vi "Barcode read.vi"(8 "error in":errorcluster, 11 "queue in":refnum<queue>) -> (0 "error out":errorcluster, 1 "exit":bool, 2 "read buffer":string, 3 "queue Out 2":refnum<queue>, 4 "Barcode Scan Bit":bool)   [LabVIEW 2015]
uses:
  Test  enqueue/AutoTest seq.ctl
  <vilib>/Utility/error.llb/whitespace.ctl
  <vilib>/Instr/_visa.llb/VISA Configure Serial Port (Instr).vi
  Galobal variable_TI.vi
  Project Setup/Globle Variable/GR_Servo.vi
panel:
  out "x = y?":bool
  out "substring":string
  out "error out 2":errorcluster
  out "error out":errorcluster
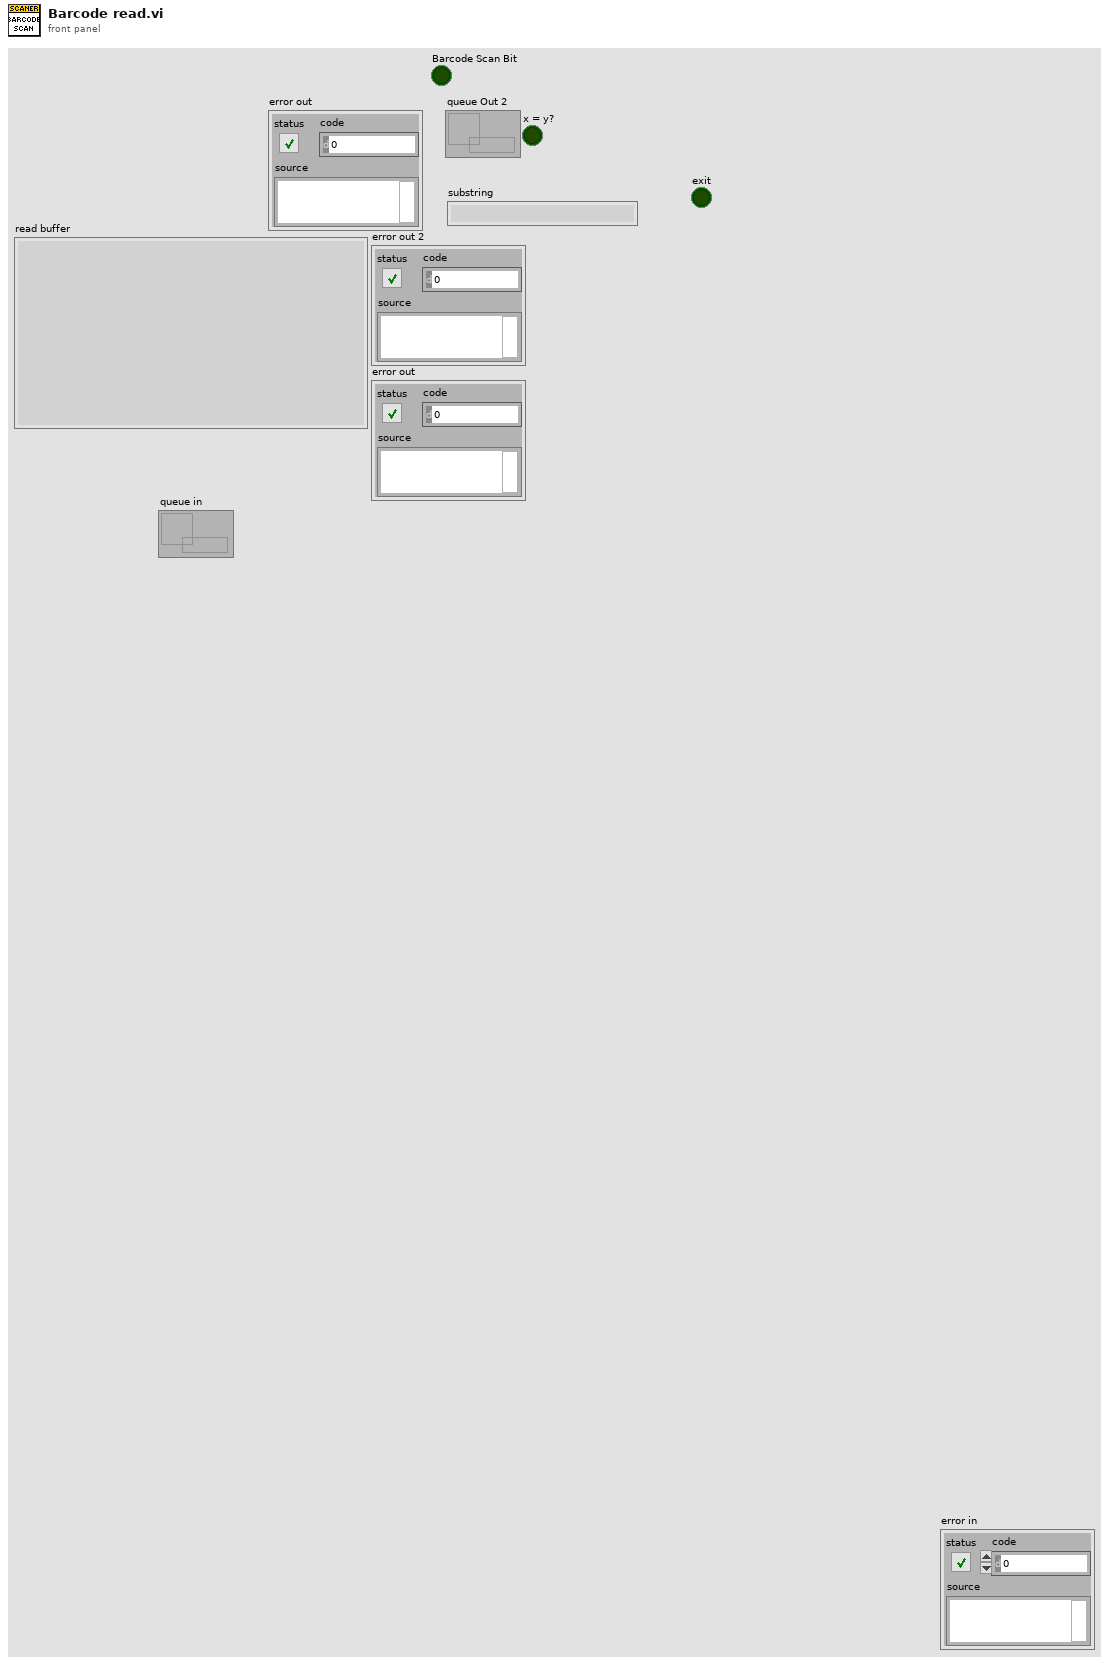
[diagram p1: front panel]
types:
  T1 = typedef "whitespace.ctl" = u16
  T2 = cluster{"MaxLoad(N) ":dbl, "Min Load(N)":dbl, "Load Offset":dbl, "Model":string, "MIC Code":string, "Dial Speedo":string, "Dial RMP":string, "Blinker":string, "Telltale":string}
  T3 = cluster{"Start":bool, "Emergency ":bool, "Reset":bool, "Home":bool, "Safety":bool}
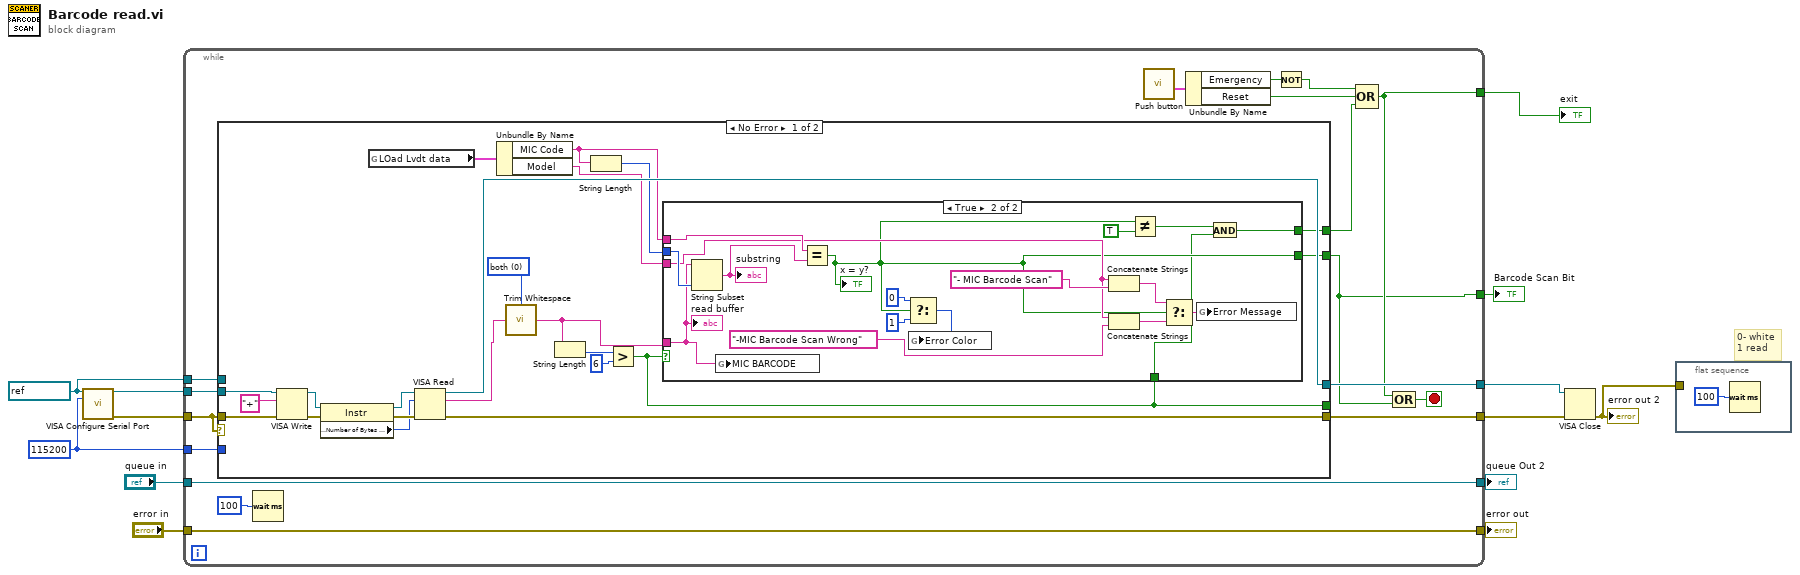
[diagram p0: block diagram]
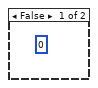
[diagram p2: hidden frame]
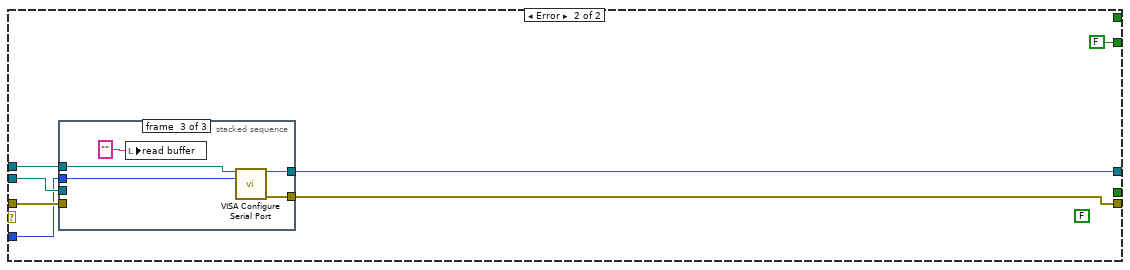
[diagram p3: hidden frame]
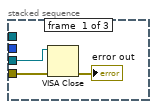
[diagram p4: hidden frame]
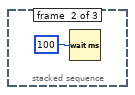
[diagram p5: hidden frame]
diagram:
  w8 = u32 115200 ("baud rate (9600)")
  w9 = refnum<visa-resource-name> "COM1" ("VISA resource name")
  # "0- white\n1 read"
  n1 = call-poly "VISA Configure Serial Port"("VISA resource name"=w9, "baud rate (9600)"=w8) -> ("VISA resource name out"=w13:refnum<visa-resource-name>, "error out"=w12:errorcluster)  [unwired: 12 in]
  n2 = while {
    tunnel: w13 -> [w30]
    tunnel: w12 -> [w28]
    tunnel: [w17] -> w11
    tunnel: [w29] -> w10
    tunnel: w9 -> [w27]
    tunnel: w8 -> [w26]
    tunnel: [w15] -> w7
    tunnel: [w23] -> w5
    tunnel: "queue in" -> [w23]
    tunnel: "error in" -> [w22]
    tunnel: [w22] -> w3
    tunnel: [w14] -> w1
    stop <- w24 stop-if-true
    n3 = case shown="No Error" w28 {
      tunnel: w30 -> [w52 w77]
      tunnel: w28 -> [w51 w76]
      tunnel: [w50 w73] -> w17
      tunnel: [w49 w72] -> w29
      tunnel: w27 -> [_ w75]
      tunnel: w26 -> [_ w74]
      tunnel: [w37 FALSE] -> w14
      tunnel: [w31 _] -> _
      tunnel: [w32 _] -> w16
      frame No Error {
        w34 = T1 0 items=["both", "start of string", "end of string"] ("location (both)")
        n4 = VISA Write(VISA resource name=w52, write buffer="+", error in (no error)=w51) -> (VISA resource name out=w47:refnum<visa-resource-name>, error out=w48:errorcluster)  [unwired: 1 out]
        n5 = property class="Instr"(reference=w47, error in=w48) -> (reference out=w46:refnum<visa-resource-name>, error out=w45:errorcluster, "Serial Settings:Number of Bytes at Serial Port"=w44:u32)
        n6 = global read "Galobal variable_TI.vi" "LOad Lvdt data"() -> (w41:T2)
        n7 = VISA Read(VISA resource name=w46, byte count=w44, error in (no error)=w45) -> (VISA resource name out=w50:refnum<visa-resource-name>, read buffer=w35:string, error out=w49:errorcluster)  [unwired: 1 out]
        n8 = Unbundle By Name(w41) -> ("MIC Code"=w40:string, "Model"=w38:string)
        n9 = call <vilib>:"Trim Whitespace.vi"("string"=w35, "location (both)"=w34) -> ("trimmed string"=w33:string)
        n10 = String Length(string=w33) -> (length=w43:i32)
        n11 = String Length(string=w40) -> (length=w39:i32)
        n12 = Greater?(x=w43, y=6) -> (0:w31:bool)
        n13 = case shown="True" w31 {
          tunnel: w33 -> [_ w58]
          tunnel: w40 -> [_ w69]
          tunnel: w39 -> [_ w70]
          tunnel: w38 -> [_ w60]
          tunnel: [_ w57] -> w37
          tunnel: w31 -> [_ w54]
          tunnel: [_ w53] -> w32
          frame False {
            (unwired) 0 ("f")
          }
          frame True {
            n14 = String Subset(string=w58, length (rest)=w70) -> (substring=w68:string)  [unwired: 1 in]
            "substring" <- w68
            n15 = global write "Galobal variable_TI.vi" "MIC BARCODE"(w58) -> ()
            n16 = Equal?(x=w69, y=w68) -> (x = y?=w57:bool)
            "x = y?" <- w57
            n17 = Select(t=0, s=w57, f=1) -> (s? t:f=w65:i32)
            n18 = global write "GR_Servo.vi" "Error Color"(w65) -> ()
            n19 = Concatenate Strings(w60, "- MIC Barcode Scan" ("string")) -> (w63:string)
            n20 = Concatenate Strings(w60, "-MIC Barcode Scan Wrong" ("string")) -> (w62:string)
            n21 = Not Equal?(x=w57, y=TRUE) -> (x != y?=w55:bool)
            n22 = Select(t=w63, s=w57, f=w62) -> (s? t:f=w61:string)
            n23 = global write "GR_Servo.vi" "Error Message"(w61) -> ()
            n24 = And(x=w55, y=w54) -> (x .and. y?=w53:bool)
            "read buffer" <- w58
          }
        }
      }
      frame Error {
        (unwired) FALSE
        n25 = stacked-sequence {
          tunnel: w77 -> [w79 _ _]
          tunnel: w76 -> [w78 _ _]
          tunnel: w75 -> [_ _ w86]
          tunnel: w74 -> [_ _ w85]
          tunnel: [_ _ w84] -> w73
          tunnel: [_ _ w83] -> w72
          frame #0 {
            n26 = VISA Close(VISA resource name=w79, error in (no error)=w78) -> (error out=→"error out":errorcluster)
          }
          frame #1 {
            n27 = Wait (ms)(milliseconds to wait=u32 100) -> ()  [unwired: 1 out]
          }
          frame #2 {
            n28 = local write "read buffer"("" ("read buffer")) -> ()
            n29 = call-poly "VISA Configure Serial Port"("VISA resource name"=w86, "baud rate (9600)"=w85) -> ("VISA resource name out"=w84:refnum<visa-resource-name>, "error out"=w83:errorcluster)  [unwired: 12 in]
          }
        }
      }
    }
    n30 = Wait (ms)(milliseconds to wait=u32 100) -> ()  [unwired: 1 out]
    n31 = call "Push button.vi"() -> ("Push Button"=w21:T3)  [unwired: 9 in, 2 out]
    n32 = Unbundle By Name(w21) -> ("Emergency"=w20:bool, "Reset"=w18:bool)
    n33 = Not(x=w20) -> (.not. x?=w19:bool)
    n34 = Compound Arithmetic op=OR(w19, w18, w16) -> (w15:bool)
    n35 = Compound Arithmetic op=OR(w15, w14) -> (w24:bool)
  }
  "exit" <- w7
  "queue Out 2" <- w5
  "error out" <- w3
  "Barcode Scan Bit" <- w1
  n36 = VISA Close(VISA resource name=w11, error in (no error)=w10) -> (error out=w2:errorcluster)
  "error out 2" <- w2
  n37 = flat-sequence {
    tunnel: w2 -> [_]
    frame #0 {
      n38 = Wait (ms)(milliseconds to wait=u32 100) -> ()  [unwired: 1 out]
    }
  }
